vi "Rotate WayPt for Extra Arc.vi"(6 "Pt 0":cluster{"x":dbl, "y":dbl, "th":dbl}, 8 "Blends In":T1[](array[typedef]), 10 "Pts":cluster{"x":dbl, "y":dbl, "th":dbl}[](array[cluster]), 11 "index":i32) -> (0 "Blends Out":T1[](array[typedef]), 1 "Pt2 vertex dist":dbl, 2 "Pt0 vertex dist":dbl, 3 "Pt Out":cluster{"x":dbl, "y":dbl, "th":dbl})   [LabVIEW 2019]
uses:
  BlendType.ctl
  Globals.vi
panel:
  out "XY Graph":cluster{"X":dbl, "Y":dbl}[](graph)
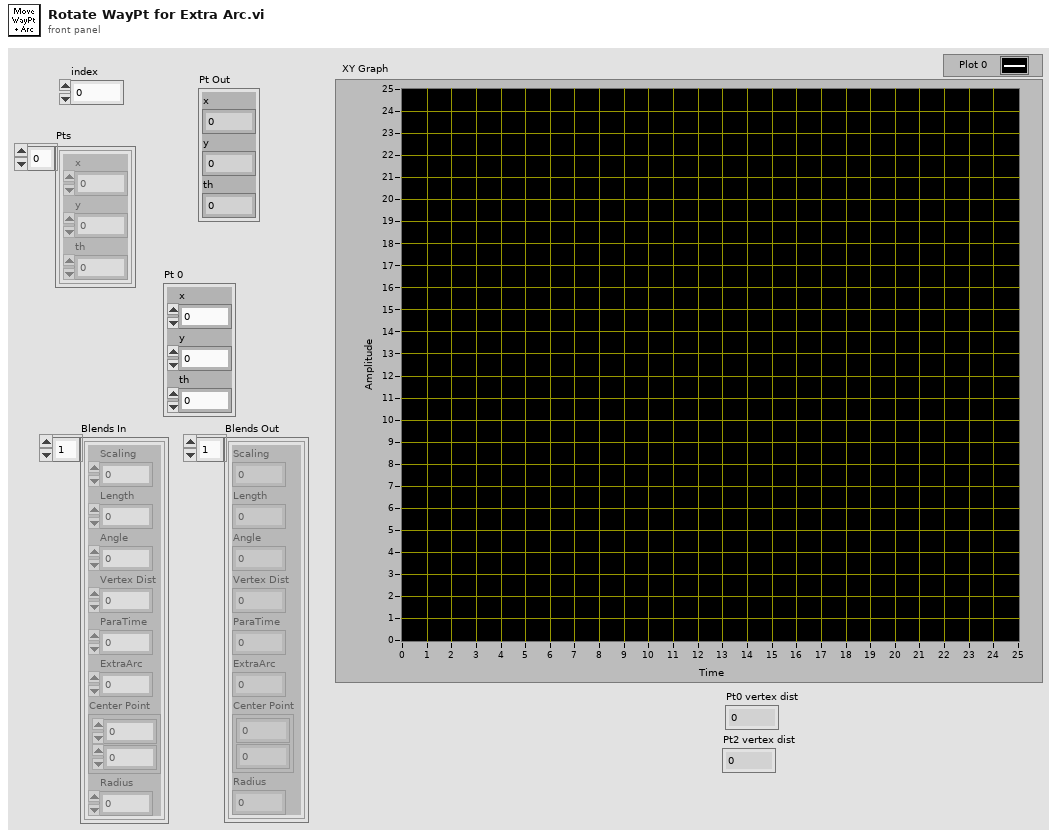
[diagram p1: front panel]
types:
  T1 = typedef "BlendType.ctl" = cluster{"Scaling":dbl, "Length":dbl, "Angle":dbl, "Vertex Dist":dbl, "ParaTime":dbl, "ExtraArc":dbl, "Center Point":cluster{dbl, dbl}, "Radius":dbl}
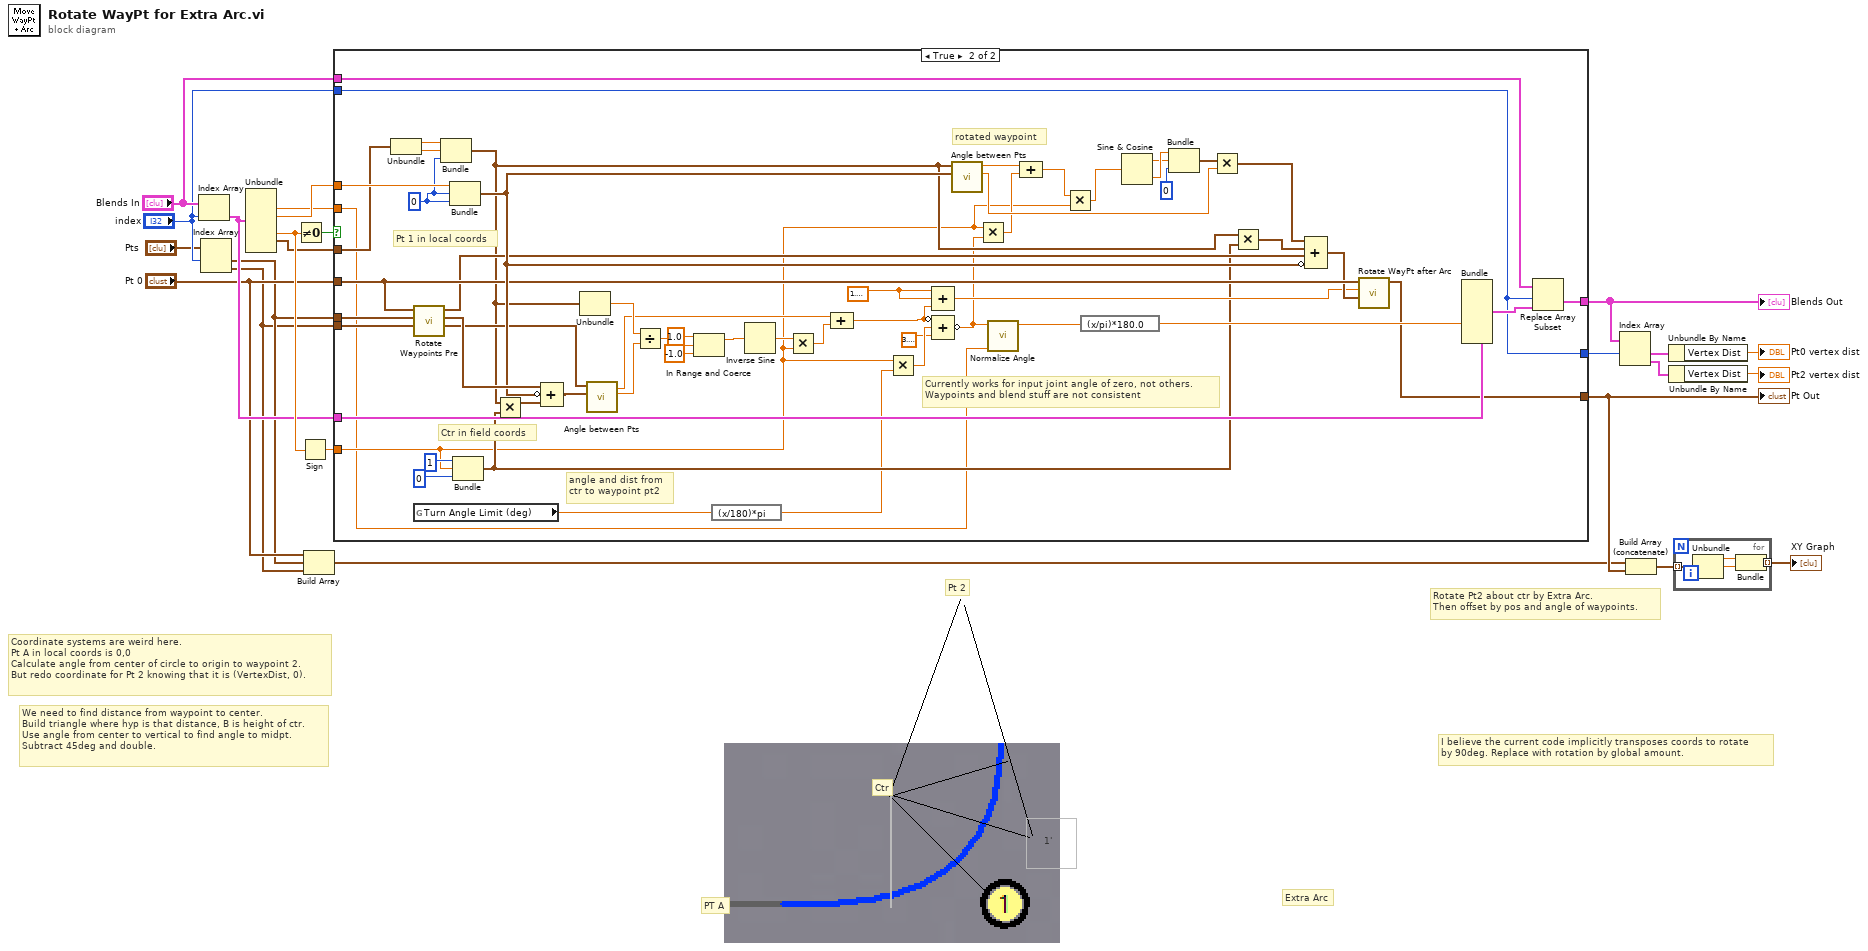
[diagram p0: block diagram]
diagram:
  # "I believe the current code implicitly transposes coords to rotate\nby 90deg. Replace with rotation by global amount."
  # "1'"
  # "We need to find distance from waypoint to center.\nBuild triangle where hyp is that distance, B is height of ctr.\nUse angle from center to vertical to find angle to midpt.\nSubtract 45deg and double."
  # "Extra Arc"
  # "Rotate Pt2 about ctr by Extra Arc.\nThen offset by pos and angle of waypoints."
  # "Ctr"
  # "Pt 2"
  # "PT A"
  # "Coordinate systems are weird here.\nPt A in local coords is 0,0\nCalculate angle from center of circle to origin to waypoint 2.\nBut redo coordinate for Pt 2 knowing that it is (VertexDist, 0)."
  n1 = Index Array(array="Blends In", index="index") -> (element=w15:T1)
  n2 = Index Array(array="Pts", index #1="index") -> (element #1=w5:cluster{"x":dbl, "y":dbl, "th":dbl}, element #2=w4:cluster{"x":dbl, "y":dbl, "th":dbl})  [unwired: 1 in]
  n3 = Unbundle(w15) -> ("Angle"=w1:dbl, "Vertex Dist"=w22:dbl, "ExtraArc"=w21:dbl, "Center Point"=w16:cluster{dbl, dbl})  [unwired: 4 out]
  n4 = Not Equal To 0?(x=w21) -> (x != 0?=w23:bool)
  n5 = Sign(1:w21) -> (0:w20:dbl)
  n6 = Build Array("Pt 0", w5, w4) -> (w3:cluster{"x":dbl, "y":dbl, "th":dbl}[])
  n7 = case shown="True" w23 {
    tunnel: w4 -> [_ w39]
    tunnel: [w26 w40] -> w17
    tunnel: w5 -> [w26 w58]
    tunnel: w15 -> [_ w76]
    tunnel: [w25 w38] -> w9
    tunnel: w22 -> [_ w71]
    tunnel: "Pt 0" -> [_ w63]
    tunnel: w20 -> [_ w45]
    tunnel: w16 -> [_ w44]
    tunnel: "Blends In" -> [w25 w43]
    tunnel: "index" -> [w24 w41]
    tunnel: [w24 w41] -> w8
    tunnel: w1 -> [_ w31]
    frame False {
    }
    frame True {
      w34 = 1.5707963267948966
      w70 = 0
      # "rotated waypoint"
      # "angle and dist from\nctr to waypoint pt2"
      # "Pt 1 in local coords"
      # "Currently works for input joint angle of zero, not others.\nWaypoints and blend stuff are not consistent"
      # "Ctr in field coords"
      n8 = Unbundle(w44) -> (w73:dbl, w72:dbl)
      n9 = call "Rotate Waypoints Pre.vi"("Pt 2"=w39, "Pt 1"=w58, "Pt 0"=w63) -> ("Pt 2 out"=w66:cluster{dbl, dbl, dbl}, "Pt 1 out"=w69:cluster{"Vertex Dist":dbl, dbl, dbl}, "Pt 1 rel to Pt0"=w61:cluster{"Vertex Dist":dbl, dbl, dbl})  [unwired: 6 in]
      n10 = global read "Globals.vi" "Turn Angle Limit (deg)"() -> (w37:dbl)
      n11 = Bundle(w73, w72, w70) -> (w50:cluster{dbl, dbl, i32})  [unwired: 1 in]
      n12 = Bundle("Vertex Dist"=w71, w70, w70) -> (w68:cluster{"Vertex Dist":dbl, i32, i32})  [unwired: 1 in]
      n13 = Bundle(1, w45, 0) -> (w46:cluster{i32, dbl, i32})  [unwired: 1 in]
      n14 = Multiply(x=w50, y=w46) -> (x*y=w49:cluster{dbl, dbl, i32})
      n15 = Compound Arithmetic op=ADD(w69, invert w68, w49) -> (w67:cluster{dbl, dbl, dbl})
      n16 = Unbundle(w50) -> (w77:dbl)  [unwired: 2 out]
      n17 = call "Angle between Pts.vi"("Pt 2"=w67, "Pt 1"=w66) -> ("Distance ft"=w65:dbl, "Angle rad"=w64:dbl)  [unwired: 8 in]
      n18 = Divide(x=w77, y=w65) -> (x/y=w30:dbl)
      n19 = In Range and Coerce(upper limit=1.0, x=w30, lower limit=-1.0) -> (coerced(x)=w29:dbl)  [unwired: 1 out]
      n20 = expression code="(x/180)*pi" ("radians to degrees")(w37) -> (w36:dbl)
      n21 = Inverse Sine(1:w29) -> (0:w56:dbl)
      n22 = Multiply(x=w56, y=w45) -> (x*y=w55:dbl)
      n23 = Compound Arithmetic op=ADD(w64, w55) -> (w74:dbl)
      n24 = Multiply(x=w45, y=w36) -> (x*y=w60:dbl)
      n25 = Compound Arithmetic op=ADD(w34, w34, w74) -> (w59:dbl)
      n26 = Compound Arithmetic op=ADD(invert w74, w60, 3.141592653589793) -> (invert w33:dbl)
      n27 = call "Angle between Pts.vi"("Pt 2"=w68, "Pt 1"=w50) -> ("Distance ft"=w78:dbl, "Angle rad"=w83:dbl)  [unwired: 8 in]
      n28 = Multiply(x=w45, y=w33) -> (x*y=w57:dbl)
      n29 = call "Normalize Angle.vi"("Initial Angle"=w31, "Angle in r"=w33) -> ("Angle out r"=w32:dbl)  [unwired: 9 in]
      n30 = Compound Arithmetic op=ADD(w83, w57) -> (w54:dbl)
      n31 = Multiply(x=w54, y=w45) -> (x*y=w53:dbl)
      n32 = expression code="(x/pi)*180.0" ("radians to degrees")(w32) -> (w75:dbl)
      n33 = Sine & Cosine(0:w53) -> (1:w80:dbl, 2:w81:dbl)
      n34 = Bundle(w81, w80, 0) -> (w79:cluster{dbl, dbl, i32})  [unwired: 1 in]
      n35 = Multiply(x=w79, y=w78) -> (x*y=w51:cluster{dbl, dbl, dbl})
      n36 = Multiply(x=w50, y=w46) -> (x*y=w52:cluster{dbl, dbl, i32})
      n37 = Compound Arithmetic op=ADD(w51, w52, w61, invert w68) -> (w62:cluster{dbl, dbl, dbl})
      n38 = call "Rotate WayPt after Arc.vi"("Phantom Waypoint"=w62, "Waypoint Line rad"=w59, "Pt 0"=w63) -> ("Phantom Waypoint out"=w40:cluster{"x":dbl, "y":dbl, "th":dbl})  [unwired: 8 in]
      n39 = Bundle(cluster=w76, "ExtraArc"=w75) -> (w42:T1)  [unwired: 7 in]
      n40 = Replace Array Subset(array=w43, new element=w42, index=w41) -> (w38:T1[])
    }
  }
  "Pt Out" <- w17
  "Blends Out" <- w9
  n41 = Index Array(array=w9, index #1=w8) -> (element #1=w13:T1, element #2=w12:T1)  [unwired: 1 in]
  n42 = Build Array (concatenate)(w3, w17) -> (w19:cluster{"x":dbl, "y":dbl, "th":dbl}[])
  n43 = Unbundle By Name(w13) -> ("Vertex Dist"=→"Pt0 vertex dist":dbl)
  n44 = Unbundle By Name(w12) -> ("Vertex Dist"=→"Pt2 vertex dist":dbl)
  n45 = for {
    tunnel: w19 -> [w85] mode=indexing
    tunnel: [w84] -> w18 mode=indexing
    n46 = Unbundle(w85) -> ("x"=w87:dbl, "y"=w86:dbl)  [unwired: 1 out]
    n47 = Bundle("x"=w87, "y"=w86) -> (w84:cluster{"x":dbl, "y":dbl})  [unwired: 1 in]
  }
  "XY Graph" <- w18
